vi "sat.vi"(2 "error in (no error)":errorcluster, 3 "x":dbl) -> (0 "error out":errorcluster, 1 "sat(x)":dbl)   [LabVIEW 2021]
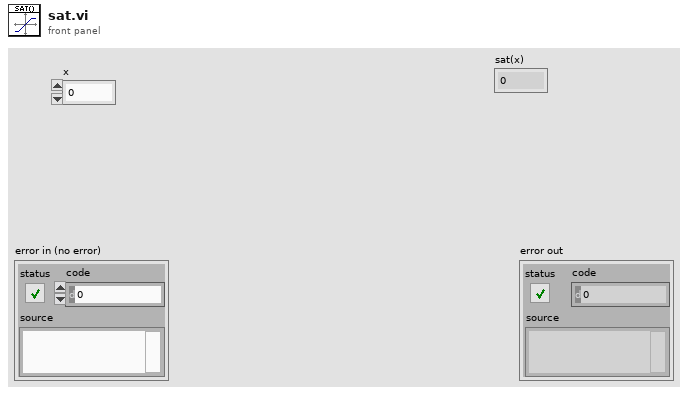
[diagram p1: front panel]
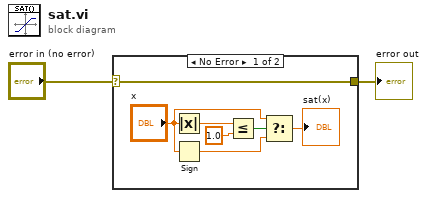
[diagram p0: block diagram]
diagram:
  n1 = case shown="No Error" "error in (no error)" {
    selector: "error in (no error)" -> [w5 w10]
    tunnel: [w5 w10] -> w1
    frame No Error {
      n2 = Absolute Value(x="x") -> (abs(x)=w4:dbl)
      n3 = Sign(1:"x") -> (0:w7:dbl)
      n4 = Less Or Equal?(x=w4, y=1.0) -> (x <= y?=w9:bool)
      n5 = Select(t="x", s=w9, f=w7) -> (s? t:f=→"sat(x)":dbl)
    }
    frame Error {
    }
  }
  "error out" <- w1
